vi "MALTCON maint status.vi"() -> ()   [LabVIEW 2018]
uses:
  <instrlib>/AltonTech MALT/AltonTech MALT200817.lvlib
panel:
  out "Local Port":u16
  in  "Address":i32=1
  out "Maintenance Requied":bool
  in  "stop":bool
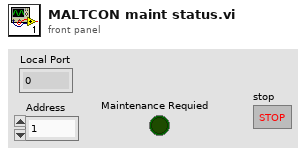
[diagram p1: front panel]
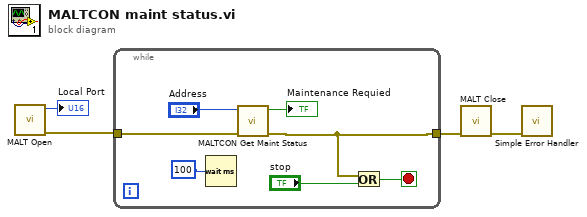
[diagram p0: block diagram]
diagram:
  n1 = call <instrlib>:"MALT Open.vi"() -> ("error out"=w4:errorcluster, "Local Port"=→"Local Port":u16)  [unwired: 10 in]
  n2 = while {
    tunnel: w4 -> [w8]
    tunnel: [w9] -> w3
    stop <- w10 stop-if-true
    n3 = Wait (ms)(milliseconds to wait=u32 100 ("millisecond timer value")) -> ()  [unwired: 1 out]
    n4 = call <instrlib>:"MALTCON Get Maint Status.vi"("error in"=w8, "Address"="Address") -> ("error out"=w9:errorcluster, "Status"=→"Maintenance Requied":bool)  [unwired: 8 in]
    n5 = Or(x=w9, y="stop") -> (x .or. y?=w10:bool)
  }
  n6 = call <instrlib>:"MALT Close.vi"("error in"=w3) -> ("error out"=w2:errorcluster)  [unwired: 10 in]
  n7 = call <vilib>:"Simple Error Handler.vi"("error in (no error)"=w2) -> ()  [unwired: 4 in, 5 out]
